vi "Shift_Value_CH0_calibration_Rev01.vi"(0 "IN1 Shift Val1":dbl, 1 "IN1 Shift Val2":dbl, 2 "Range IN1":dbl, 3 "USB Interface Name":refnum<visa-resource-name>="COM3", 4 "Input buffer size":u32=16384, 5 "error in (no error)":errorcluster, 9 "WRITE":bool, 19 "Sign Value":dbl) -> (6 "MB address":string, 7 "MB value":u8 format="%x", 8 "UB address":string, 10 "HB address":string, 11 "error out":errorcluster, 12 "LB address":string, 13 "UB value":u8 format="%x", 14 "IN1 shift value uV":dbl, 15 "IN1 shift val HEX uV":u32 format="%x", 16 "Sign Addrss":string, 17 "HB value":u8 format="%x", 18 "LB value":u8 format="%x")   [LabVIEW 2012]
panel:
  out "LB value":string
  out "HB value":string
  out "UB value":string
  out "MB value":string
  # "1. Computes address based on the input range \"Range IN\"\n2. Take absolute values of positive and negative voltage reads in uV compares them and subtracts smaller value from the larger one. The result is devided by 2.\nIf VAL1>VAL2: ( |VAL1| - |VAL2| )/ 2"
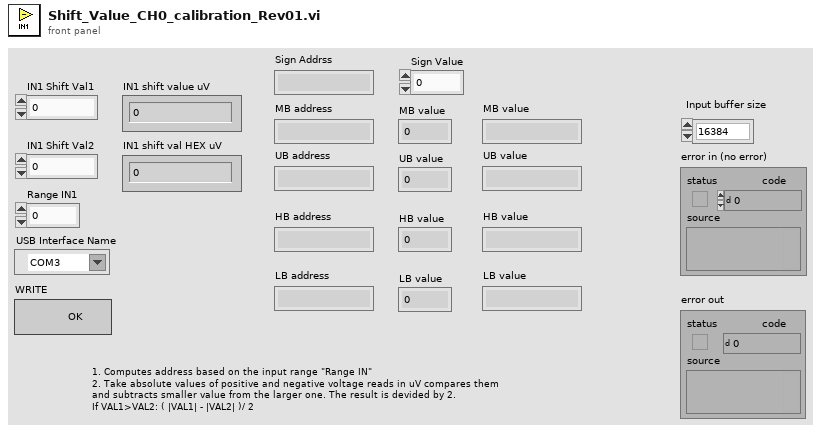
[diagram p1: front panel]
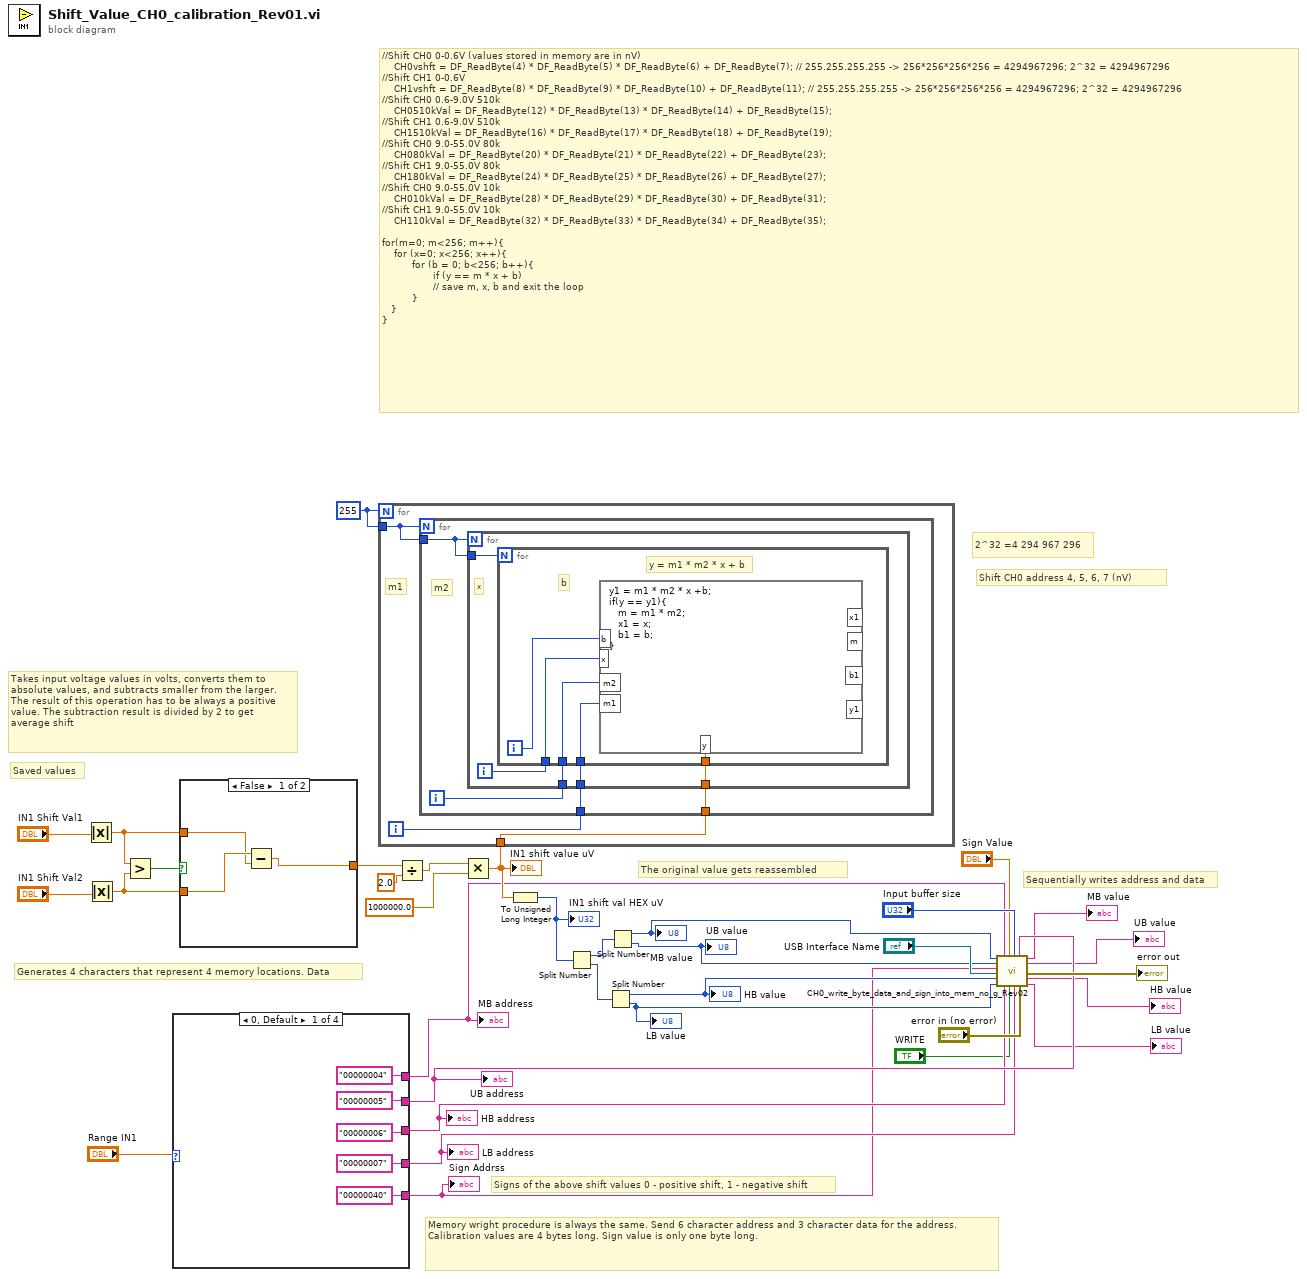
[diagram p0: block diagram]
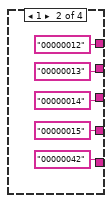
[diagram p2: hidden frame]
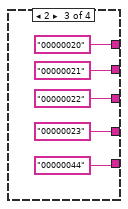
[diagram p3: hidden frame]
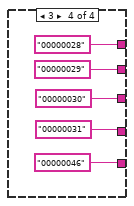
[diagram p4: hidden frame]
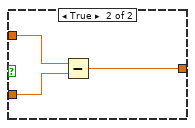
[diagram p5: hidden frame]
diagram:
  w4 = 255
  # "Shift CH0 address 4, 5, 6, 7 (nV)"
  # "Signs of the above shift values 0 - positive shift, 1 - negative shift"
  # "The original value gets reassembled"
  # "//Shift CH0 0-0.6V (values stored in memory are in nV)     \n    CH0vshft = DF_ReadByte(4) * DF_ReadByte(5) * DF_ReadByte(6) + DF_ReadByte(7); // 255.255.255.255 -> 256*256*256*256 = 4294967296; 2^32 = 4294967296\n//Shift CH1 0-0.6V\n    CH1vshft = DF_ReadByte(8) * DF_ReadByte(9) * DF_ReadByte(10) + DF_ReadByte(11); // 255.255.255.255 -> 256*256*256*256 = 4294967296; 2^32 = 4294967296\n//Shift CH0 0.6-9.0V 510k\n    CH0510kVal = DF_ReadByte(12) * DF_ReadByte(13) * DF_ReadByte(14) + DF_ReadByte(15);\n//Shift CH1 0.6-9.0V 510k\n    CH1510kVal = DF_ReadByte(16) * DF_ReadByte(17) * DF_ReadByte(18) + DF_ReadByte(19);\n//Shift CH0 9.0-55.0V 80k            \n    CH080kVal = DF_ReadByte(20) * DF_ReadByte(21) * DF_ReadByte(22) + DF_ReadByte(23);\n//Shift CH1 9.0-55.0V 80k\n    CH180kVal = DF_ReadByte(24) * DF_ReadByte(25) * DF_ReadByte(26) + DF_ReadByte(27);\n//Shift CH0 9.0-55.0V 10k\n    CH010kVal = DF_ReadByte(28) * DF_ReadByte(29) * DF_ReadByte(30) + DF_ReadByte(31);\n//Shift CH1 9.0-55.0V 10k\n    CH110kVal = DF_ReadByte(32) * DF_ReadByte(33) * DF_ReadByte(34) + DF_ReadByte(35);\n\nfor(m=0; m<256; m++){\n    for (x=0; x<256; x++){\n          for (b = 0; b<256; b++){\n                 if (y == m * x + b)\n                 // save m, x, b and exit the loop\n          }\n   }\n}"
  # "Saved values"
  # "Sequentially writes address and data"
  # "Memory wright procedure is always the same. Send 6 character address and 3 character data for the address.\nCalibration values are 4 bytes long. Sign value is only one byte long."
  # "2^32 =4 294 967 296"
  # "Generates 4 characters that represent 4 memory locations. Data"
  # "Takes input voltage values in volts, converts them to absolute values, and subtracts smaller from the larger. The result of this operation has to be always a positive value. The subtraction result is divided by 2 to get average shift"
  n1 = Absolute Value(x="IN1 Shift Val1") -> (abs(x)=w31:dbl)
  n2 = Absolute Value(x="IN1 Shift Val2") -> (abs(x)=w30:dbl)
  n3 = Greater?(x=w31, y=w30) -> (0:w32:bool)
  n4 = case shown="0, Default" "Range IN1" {
    tunnel: ["00000004" "00000012" "00000020" "00000028"] -> w1
    tunnel: ["00000005" "00000013" "00000021" "00000029"] -> w15
    tunnel: ["00000006" "00000014" "00000022" "00000030"] -> w14
    tunnel: ["00000007" "00000015" "00000023" "00000031"] -> w12
    tunnel: ["00000040" "00000042" "00000044" "00000046"] -> w6
    frame 0, Default {
    }
    frame 1 {
    }
    frame 2 {
    }
    frame 3 {
    }
  }
  "MB address" <- w1
  "UB address" <- w15
  "HB address" <- w14
  "LB address" <- w12
  "Sign Addrss" <- w6
  n5 = case shown="False" w32 {
    tunnel: w31 -> [w56 w60]
    tunnel: w30 -> [w57 w59]
    tunnel: [w55 w58] -> w29
    frame False {
      n6 = Subtract(x=w57, y=w56) -> (x-y=w55:dbl)
    }
    frame True {
      n7 = Subtract(x=w60, y=w59) -> (x-y=w58:dbl)
    }
  }
  n8 = Divide(x=w29, y=2.0) -> (x/y=w27:dbl)
  n9 = Multiply(x=w27, y=1000000.0) -> (x*y=w3:dbl)
  "IN1 shift value uV" <- w3
  n10 = for {
    N: w4 -> [_]
    tunnel: w4 -> [w63]
    tunnel: w3 -> [w61]
    i -> [w62]
    # "m1"
    n11 = for {
      N: w63 -> [_]
      tunnel: w63 -> [w67]
      tunnel: w62 -> [w66]
      tunnel: w61 -> [w64]
      i -> [w65]
      # "m2"
      n12 = for {
        N: w67 -> [_]
        tunnel: w67 -> [w72]
        tunnel: w66 -> [w71]
        tunnel: w65 -> [w70]
        tunnel: w64 -> [w68]
        i -> [w69]
        # "x"
        n13 = for {
          N: w72 -> [_]
          tunnel: w71 -> [w77]
          tunnel: w70 -> [w76]
          tunnel: w69 -> [w75]
          tunnel: w68 -> [w73]
          i -> [w74]
          # "y = m1 * m2 * x + b"
          # "b"
          n14 = formula code="y1 = m1 * m2 * x +b;\nif(y == y1){\n   m = m1 * m2;\n   x1 = x;\n   b1 = b;\n}"("m1"=w77, "m2"=w76, "x"=w75, "b"=w74, "y"=w73) -> ()  [unwired: 4 out]
        }
      }
    }
  }
  n15 = To Unsigned Long Integer(number=w3) -> (unsigned 32bit integer=w25:u32)
  "IN1 shift val HEX uV" <- w25
  n16 = Split Number(x=w25) -> (hi(x)=w24:u16, lo(x)=w23:u16)
  n17 = Split Number(x=w23) -> (hi(x)=w17:u8, lo(x)=w16:u8)
  "HB value" <- w17
  "LB value" <- w16
  n18 = Split Number(x=w24) -> (hi(x)=w2:u8, lo(x)=w18:u8)
  "MB value" <- w2
  "UB value" <- w18
  n19 = call "CH0_write_byte_data_and_sign_into_mem_no_g_Rev02.vi"("MB data"=w2, "UB data"=w18, "Sign addrss 8 byte"=w6, "USB Interface Name"="USB Interface Name", "HB data"=w17, "LB data"=w16, "MB addrss 8 byte"=w1, "HB addrss 8 byte"=w14, "Sign data 3 byte"="Sign Value", "WRITE DATA"="WRITE", "Input buffer size"="Input buffer size", "LB addrss 8 byte"=w12, "UB addrss 8 byte"=w15, "error in (no error)"="error in (no error)") -> ("MB data 3 byte"=→"MB value":string, "UB data 3 byte"=→"UB value":string, "error out"=→"error out":errorcluster, "HB data 3 byte"=→"HB value":string, "LB data 3 byte"=→"LB value":string)  [unwired: 1 in]
